vi "pf_reverse_3Dprofile.vi"(8 "error in (no error)":errorcluster, 10 "Peak in":sgl, 11 "IMAQ Session in":refnum<k11>) -> (0 "error out":errorcluster, 2 "Peak out":sgl, 3 "IMAQ Session out":refnum<k11>)   [LabVIEW 2025, in "Photonfocus_Toolkit.lvlib"]
uses:
  Photonfocus_Toolkit.lvlib
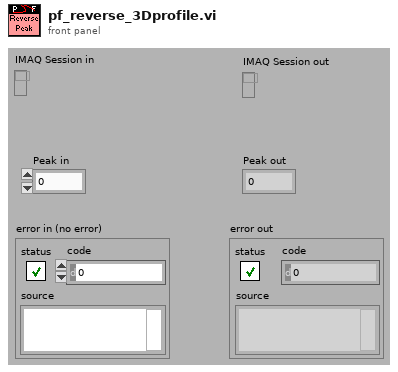
[diagram p1: front panel]
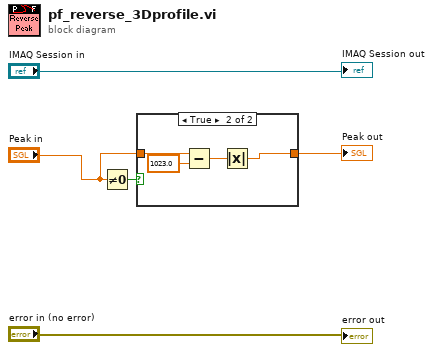
[diagram p0: block diagram]
diagram:
  n1 = Not Equal To 0?(x="Peak in") -> (x != 0?=w4:bool)
  n2 = case shown="True" w4 {
    tunnel: "Peak in" -> [w6 w10]
    tunnel: [w6 w7] -> w2
    frame False {
    }
    frame True {
      n3 = Subtract(x=w10, y=sgl 1023.0) -> (x-y=w8:sgl)
      n4 = Absolute Value(x=w8) -> (abs(x)=w7:sgl)
    }
  }
  "Peak out" <- w2
  "error out" <- "error in (no error)"
  "IMAQ Session out" <- "IMAQ Session in"
